vi "Update Value.vi"(6 "Time":dbl, 8 "error in (no error)":errorcluster, 11 "2WayValve in":refnum<class "2WayValve.lvclass">) -> (0 "error out":errorcluster, 1 "Update":bool, 2 "Value":variant, 3 "2WayValve out":refnum<class "2WayValve.lvclass">)   [LabVIEW 2020, in "VolatusGUI.lvlib" / "2WayValve.lvclass"]
uses:
  2WayValve.lvclass
  2WayValve.lvclass/2WayValve.ctl
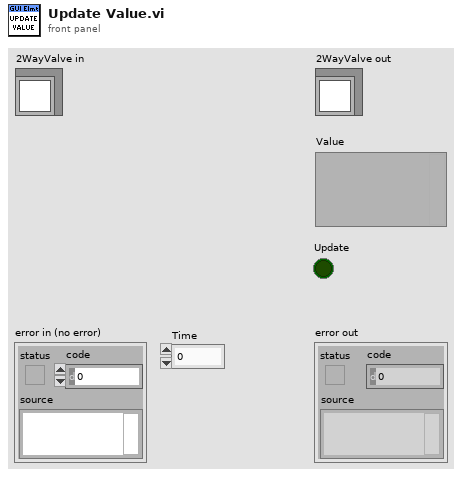
[diagram p1: front panel]
types:
  T1 = typedef "VolatusGUI.lvlib/2WayValve.lvclass/Values.ctl" = cluster{"Command":T2, "CmdFB":T2, "Closed":T2, "Open":T2, "Energized":T2}
  T2 = typedef "VolatusGUI.lvlib/2WayValve.lvclass/Channel State.ctl" = cluster{"Value":bool, "Stale":bool, "Config":bool, "Error":bool, "Prev":bool}
  T3 = typedef "VolatusGUI.lvlib/2WayValve.lvclass/Unused Element.ctl" = cluster{"Command":bool, "Feedback":bool, "Energized":bool}
  T4 = typedef "VolatusGUI.lvlib/2WayValve.lvclass/Valve Pictures.ctl" = cluster{"Command":T5, "Feedback":T7, "Energized":T8}
  T5 = typedef "VolatusGUI.lvlib/2WayValve.lvclass/Command Pictures.ctl" = cluster{"Error":T6, "Config":T6, "Stale":T6, "Close":T6, "Open":T6, "TranClose":T6, "TranOpen":T6}
  T6 = typedef "VolatusGUI.lvlib/2WayValve.lvclass/Picture.ctl" = enum16{"Blank", "OutClose", "OutOpen", "OutTranClose", "OutTranOpen", "OutConfig", "OutStale", "OutError", "InClose", "InOpen", "InTranClose", "InTranOpen", "InConfig", "InStale", "InError", "EnOff", "EnOn", "EnConfig", "EnStale", "EnError"}
  T7 = typedef "VolatusGUI.lvlib/2WayValve.lvclass/Feedback Pictures.ctl" = cluster{"Error":T6, "Config":T6, "Stale":T6, "Closed":T6, "Open":T6, "TranClose":T6, "TranOpen":T6}
  T8 = typedef "VolatusGUI.lvlib/2WayValve.lvclass/Energized Pictures.ctl" = cluster{"Error":T6, "Config":T6, "Stale":T6, "False":T6, "True":T6}
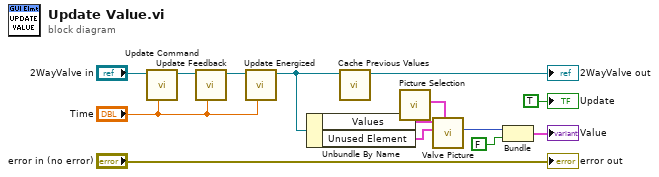
[diagram p0: block diagram]
diagram:
  n1 = call "Update Command.vi"("Time"="Time", "2WayValve in"="2WayValve in") -> ("2WayValve out"=w12:refnum<class "2WayValve.lvclass">)  [unwired: 8 in, 1 out]
  n2 = call "Update Feedback.vi"("Time"="Time", "2WayValve in"=w12) -> ("2WayValve out"=w11:refnum<class "2WayValve.lvclass">)  [unwired: 8 in, 1 out]
  n3 = call "Update Energized.vi"("Time"="Time", "2WayValve in"=w11) -> ("2WayValve out"=w9:refnum<class "2WayValve.lvclass">)  [unwired: 8 in, 1 out]
  n4 = Unbundle By Name(w9) -> ("Values"=w6:T1, "Unused Element"=w8:T3)
  n5 = call "Cache Previous Values.vi"("2WayValve in"=w9) -> ("2WayValve out"=→"2WayValve out":refnum<class "2WayValve.lvclass">)  [unwired: 9 in, 1 out]
  n6 = call "Picture Selection.vi"() -> ("Valve Pictures"=w7:T4)  [unwired: 11 in]
  n7 = call "Valve Picture.vi"("Valve Pictures"=w7, "Unused Element"=w8, "Values"=w6) -> ("Valve Picture"=w5:picture)  [unwired: 8 in]
  n8 = Bundle("Valve Picture"=w5, FALSE) -> (→"Value":cluster{"Valve Picture":picture, bool})  [unwired: 1 in]
  "error out" <- "error in (no error)"
  "Update" <- TRUE ("Update")
